vi "TelemetrySynchronizer.vi"() -> ()   [LabVIEW 2009]
uses:
  Api/TelemetryServer/TelemetryServer_Global.vi
panel:
  in  "TelemetryMaster":string="FringeTracker[0].CompleteControllerSet.ControllerData.ChannelData[0].CalibratedBinData[0]"
  in  "Telemetry":string="FringeTracker[0].CompleteControllerSet.ControllerData.ChannelData[0].CalibratedBinData[0]"
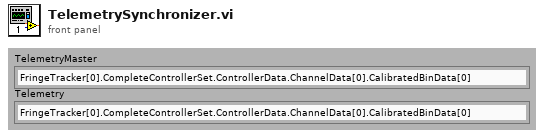
[diagram p1: front panel]
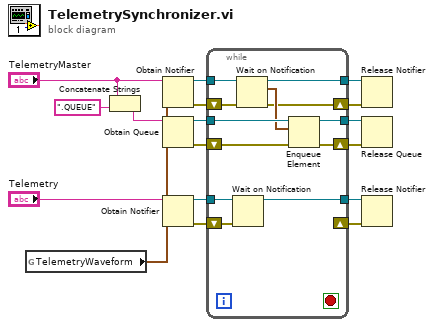
[diagram p0: block diagram]
diagram:
  n1 = global read "TelemetryServer_Global.vi" "TelemetryWaveform"() -> (w4:waveform(dbl))
  n2 = Concatenate Strings("TelemetryMaster", ".QUEUE" ("chaîne")) -> (w9:string)
  n3 = Obtain Notifier(name (unnamed)="TelemetryMaster", notification data type=w4) -> (notifier out=w16:refnum<notifier>, error out=w5:errorcluster)  [unwired: 2 in, 1 out]
  n4 = Obtain Queue(name (unnamed)=w9, element data type=w4) -> (queue out=w7:refnum<queue>, error out=w6:errorcluster)  [unwired: 3 in, 1 out]
  n5 = Obtain Notifier(name (unnamed)="Telemetry", notification data type=w4) -> (notifier out=w13:refnum<notifier>, error out=w14:errorcluster)  [unwired: 2 in, 1 out]
  n6 = while {
    tunnel: w16 -> [w29]
    shift-right: [w18] -> w3
    shift-left: w5 -> [w24]
    tunnel: [w28] -> w15
    shift-right: [_] -> w12
    shift-left: w14 -> [w27]
    tunnel: w13 -> [w26]
    tunnel: [w25] -> w11
    tunnel: w7 -> [w22]
    shift-right: [w19] -> w2
    shift-left: w6 -> [w23]
    tunnel: [w20] -> w1
    stop <- _ stop-if-true
    n7 = Wait on Notification(notifier=w26, error in (no error)=w27) -> (notifier out=w25:refnum<notifier>)  [unwired: 2 in, 3 out]
    n8 = Wait on Notification(notifier=w29, error in (no error)=w24) -> (notifier out=w28:refnum<notifier>, notification=w21:waveform(dbl), error out=w18:errorcluster)  [unwired: 2 in, 1 out]
    n9 = Enqueue Element(queue=w22, element=w21, error in (no error)=w23) -> (queue out=w20:refnum<queue>, error out=w19:errorcluster)  [unwired: 1 in, 1 out]
  }
  n10 = Release Notifier(notifier=w15, error in (no error)=w3) -> ()  [unwired: 1 in, 3 out]
  n11 = Release Queue(queue=w1, error in (no error)=w2) -> ()  [unwired: 1 in, 3 out]
  n12 = Release Notifier(notifier=w11, error in (no error)=w12) -> ()  [unwired: 1 in, 3 out]
